vi "getY.vi"(8 "error in (no error)":errorcluster, 11 "Circle in":refnum<class "Circle.lvclass">) -> (0 "error out":errorcluster, 2 "y":i32, 3 "Circle out":refnum<class "Circle.lvclass">)   [LabVIEW 2018, in "Circle.lvclass"]
uses:
  Circle.lvclass
  Circle.lvclass/Circle.ctl
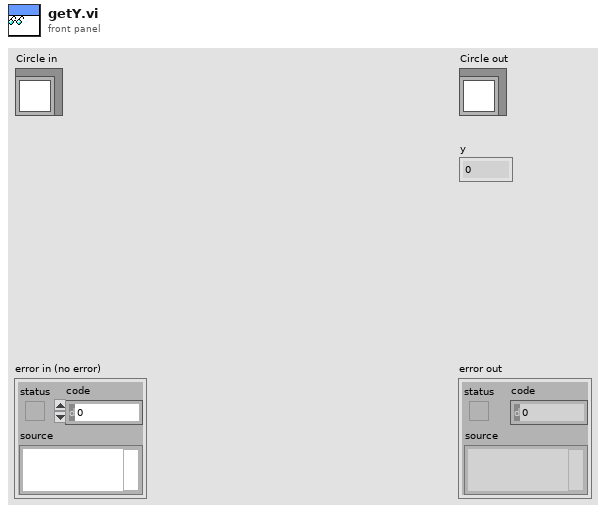
[diagram p1: front panel]
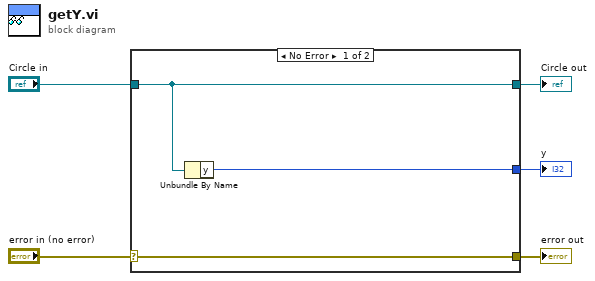
[diagram p0: block diagram]
diagram:
  n1 = case shown="No Error" "error in (no error)" {
    selector: "error in (no error)" -> [w8 w9]
    tunnel: [w8 w9] -> w4
    tunnel: [w7 w10] -> w2
    tunnel: "Circle in" -> [w7 w10]
    tunnel: [w6 _] -> w1
    frame No Error {
      n2 = Unbundle By Name(w7) -> ("y"=w6:i32)
    }
    frame Error {
    }
  }
  "error out" <- w4
  "Circle out" <- w2
  "y" <- w1
